vi "TR_DRAW_Trajectory_(offline).vi"(0 "Post-processing parameters":variant, 5 "XY data in":T1=[{"X"=300.0, "Y"=306.0}, {"X"=299.0, "Y"=306.0}, {"X"=295.0, "Y"=297.0}, {"X"=300.0, "Y"=305.0}, {"X"=300.0, "Y"=305.0}, {"X"=299.0, "Y"=306.0}, {"X"=301.0, "Y"=305.0}, {"X"=302.0, "Y"=305.0}, {"X"=299.0, "Y"=306.0}, {"X"=300.0, "Y"=305.0}, {"X"=301.0, "Y"=305.0}, {"X"=300.0, "Y"=305.0}, {"X"=296.0, "Y"=296.0}, {"X"=302.0, "Y"=305.0}, {"X"=300.0, "Y"=305.0}, {"X"=301.0, "Y"=304.0}, {"X"=301.0, "Y"=304.0}, {"X"=301.0, "Y"=304.0}, {"X"=301.0, "Y"=303.0}, {"X"=301.0, "Y"=303.0}, {"X"=301.0, "Y"=303.0}, {"X"=300.0, "Y"=303.0}, {"X"=300.0, "Y"=303.0}, {"X"=301.0, "Y"=303.0}, {"X"=301.0, "Y"=304.0}, {"X"=302.0, "Y"=304.0}, {"X"=303.0, "Y"=304.0}, {"X"=304.0, "Y"=305.0}, {"X"=305.0, "Y"=305.0}, {"X"=306.0, "Y"=305.0}, {"X"=308.0, "Y"=306.0}, {"X"=310.0, "Y"=307.0}, {"X"=311.0, "Y"=309.0}, {"X"=314.0, "Y"=310.0}, {"X"=315.0, "Y"=312.0}, {"X"=318.0, "Y"=315.0}, {"X"=319.0, "Y"=318.0}, {"X"=321.0, "Y"=321.0}, {"X"=323.0, "Y"=324.0}, {"X"=325.0, "Y"=327.0}, {"X"=326.0, "Y"=331.0}, {"X"=327.0, "Y"=335.0}, {"X"=327.0, "Y"=338.0}, {"X"=327.0, "Y"=342.0}, {"X"=326.0, "Y"=347.0}, {"X"=325.0, "Y"=351.0}, {"X"=323.0, "Y"=355.0}, {"X"=321.0, "Y"=360.0}, {"X"=320.0, "Y"=364.0}, {"X"=317.0, "Y"=368.0}, {"X"=315.0, "Y"=372.0}, {"X"=312.0, "Y"=375.0}, {"X"=310.0, "Y"=379.0}, {"X"=308.0, "Y"=382.0}, {"X"=305.0, "Y"=385.0}, {"X"=303.0, "Y"=388.0}, {"X"=299.0, "Y"=391.0}, {"X"=296.0, "Y"=395.0}, {"X"=292.0, "Y"=398.0}, {"X"=287.0, "Y"=401.0}, {"X"=283.0, "Y"=405.0}, {"X"=278.0, "Y"=408.0}, {"X"=273.0, "Y"=411.0}, {"X"=268.0, "Y"=414.0}, {"X"=264.0, "Y"=417.0}, {"X"=259.0, "Y"=419.0}, {"X"=255.0, "Y"=421.0}, {"X"=250.0, "Y"=423.0}, {"X"=246.0, "Y"=424.0}, {"X"=241.0, "Y"=425.0}, {"X"=237.0, "Y"=426.0}, {"X"=232.0, "Y"=426.0}, {"X"=227.0, "Y"=426.0}, {"X"=223.0, "Y"=425.0}, {"X"=219.0, "Y"=425.0}, {"X"=215.0, "Y"=425.0}, {"X"=211.0, "Y"=425.0}, {"X"=209.0, "Y"=425.0}, {"X"=206.0, "Y"=424.0}, {"X"=203.0, "Y"=423.0}, {"X"=200.0, "Y"=421.0}, {"X"=197.0, "Y"=420.0}, {"X"=193.0, "Y"=417.0}, {"X"=189.0, "Y"=414.0}, {"X"=185.0, "Y"=411.0}, {"X"=180.0, "Y"=408.0}, {"X"=175.0, "Y"=406.0}, {"X"=170.0, "Y"=402.0}, {"X"=166.0, "Y"=399.0}, {"X"=161.0, "Y"=395.0}, {"X"=156.0, "Y"=390.0}, {"X"=152.0, "Y"=385.0}, {"X"=148.0, "Y"=379.0}, {"X"=145.0, "Y"=373.0}, {"X"=142.0, "Y"=367.0}, {"X"=140.0, "Y"=359.0}, {"X"=137.0, "Y"=353.0}, {"X"=135.0, "Y"=346.0}, {"X"=134.0, "Y"=339.0}, {"X"=132.0, "Y"=332.0}, {"X"=131.0, "Y"=325.0}, {"X"=131.0, "Y"=318.0}, {"X"=130.0, "Y"=312.0}, {"X"=129.0, "Y"=305.0}, {"X"=128.0, "Y"=299.0}, {"X"=127.0, "Y"=293.0}, {"X"=126.0, "Y"=286.0}, {"X"=125.0, "Y"=279.0}, {"X"=123.0, "Y"=273.0}, {"X"=122.0, "Y"=266.0}, {"X"=120.0, "Y"=259.0}, {"X"=119.0, "Y"=252.0}, {"X"=117.0, "Y"=245.0}, {"X"=116.0, "Y"=239.0}, {"X"=114.0, "Y"=233.0}, {"X"=112.0, "Y"=228.0}, {"X"=111.0, "Y"=223.0}, {"X"=110.0, "Y"=217.0}, {"X"=109.0, "Y"=212.0}, {"X"=108.0, "Y"=206.0}, {"X"=107.0, "Y"=200.0}, {"X"=107.0, "Y"=194.0}, {"X"=107.0, "Y"=187.0}, {"X"=108.0, "Y"=180.0}, {"X"=109.0, "Y"=174.0}, {"X"=110.0, "Y"=167.0}, {"X"=111.0, "Y"=161.0}, {"X"=113.0, "Y"=155.0}, {"X"=115.0, "Y"=149.0}, {"X"=117.0, "Y"=142.0}, {"X"=118.0, "Y"=137.0}, {"X"=120.0, "Y"=131.0}, {"X"=122.0, "Y"=125.0}, {"X"=125.0, "Y"=120.0}, {"X"=127.0, "Y"=114.0}, {"X"=129.0, "Y"=109.0}, {"X"=132.0, "Y"=105.0}, {"X"=135.0, "Y"=100.0}, {"X"=138.0, "Y"=96.0}, {"X"=141.0, "Y"=91.0}, {"X"=145.0, "Y"=87.0}, {"X"=148.0, "Y"=84.0}, {"X"=151.0, "Y"=81.0}, {"X"=154.0, "Y"=78.0}, {"X"=156.0, "Y"=77.0}, {"X"=157.0, "Y"=75.0}, {"X"=160.0, "Y"=73.0}, {"X"=163.0, "Y"=72.0}, {"X"=165.0, "Y"=71.0}, {"X"=167.0, "Y"=70.0}, {"X"=171.0, "Y"=68.0}, {"X"=173.0, "Y"=67.0}, {"X"=176.0, "Y"=66.0}, {"X"=179.0, "Y"=65.0}, {"X"=183.0, "Y"=65.0}, {"X"=187.0, "Y"=64.0}, {"X"=191.0, "Y"=64.0}, {"X"=195.0, "Y"=64.0}, {"X"=198.0, "Y"=64.0}, {"X"=202.0, "Y"=65.0}, {"X"=205.0, "Y"=66.0}, {"X"=209.0, "Y"=67.0}, {"X"=213.0, "Y"=67.0}, {"X"=217.0, "Y"=69.0}, {"X"=221.0, "Y"=70.0}, {"X"=226.0, "Y"=72.0}, {"X"=230.0, "Y"=73.0}, {"X"=236.0, "Y"=75.0}, {"X"=240.0, "Y"=77.0}, {"X"=245.0, "Y"=79.0}, {"X"=249.0, "Y"=82.0}, {"X"=253.0, "Y"=84.0}, {"X"=258.0, "Y"=87.0}, {"X"=262.0, "Y"=89.0}, {"X"=266.0, "Y"=92.0}, {"X"=269.0, "Y"=95.0}, {"X"=274.0, "Y"=98.0}, {"X"=278.0, "Y"=101.0}, {"X"=281.0, "Y"=104.0}, {"X"=285.0, "Y"=107.0}, {"X"=289.0, "Y"=111.0}, {"X"=292.0, "Y"=115.0}, {"X"=296.0, "Y"=118.0}, {"X"=300.0, "Y"=122.0}, {"X"=303.0, "Y"=126.0}, {"X"=307.0, "Y"=130.0}, {"X"=310.0, "Y"=134.0}, {"X"=313.0, "Y"=138.0}, {"X"=316.0, "Y"=142.0}, {"X"=319.0, "Y"=146.0}, {"X"=323.0, "Y"=150.0}, {"X"=326.0, "Y"=155.0}, {"X"=329.0, "Y"=160.0}, {"X"=333.0, "Y"=165.0}, {"X"=336.0, "Y"=170.0}, {"X"=340.0, "Y"=176.0}, {"X"=343.0, "Y"=181.0}, {"X"=346.0, "Y"=186.0}, {"X"=349.0, "Y"=192.0}, {"X"=353.0, "Y"=197.0}, {"X"=356.0, "Y"=202.0}, {"X"=359.0, "Y"=208.0}, {"X"=362.0, "Y"=214.0}, {"X"=364.0, "Y"=220.0}, {"X"=367.0, "Y"=227.0}, {"X"=369.0, "Y"=234.0}, {"X"=372.0, "Y"=242.0}, {"X"=374.0, "Y"=249.0}, {"X"=375.0, "Y"=258.0}, {"X"=377.0, "Y"=266.0}, {"X"=378.0, "Y"=275.0}, {"X"=378.0, "Y"=283.0}, {"X"=379.0, "Y"=291.0}, {"X"=378.0, "Y"=298.0}, {"X"=378.0, "Y"=306.0}, {"X"=377.0, "Y"=314.0}, {"X"=375.0, "Y"=321.0}, {"X"=374.0, "Y"=329.0}, {"X"=372.0, "Y"=337.0}, {"X"=369.0, "Y"=345.0}, {"X"=366.0, "Y"=353.0}, {"X"=363.0, "Y"=361.0}, {"X"=360.0, "Y"=368.0}, {"X"=356.0, "Y"=375.0}, {"X"=353.0, "Y"=382.0}, {"X"=349.0, "Y"=388.0}, {"X"=345.0, "Y"=394.0}, {"X"=341.0, "Y"=400.0}, {"X"=337.0, "Y"=406.0}, {"X"=333.0, "Y"=411.0}, {"X"=328.0, "Y"=417.0}, {"X"=323.0, "Y"=422.0}, {"X"=318.0, "Y"=428.0}, {"X"=312.0, "Y"=433.0}, {"X"=306.0, "Y"=439.0}, {"X"=300.0, "Y"=444.0}, {"X"=293.0, "Y"=448.0}, {"X"=287.0, "Y"=453.0}, {"X"=280.0, "Y"=457.0}, {"X"=273.0, "Y"=461.0}, {"X"=268.0, "Y"=465.0}, {"X"=262.0, "Y"=468.0}, {"X"=255.0, "Y"=472.0}, {"X"=249.0, "Y"=475.0}, {"X"=242.0, "Y"=479.0}, {"X"=235.0, "Y"=482.0}, {"X"=227.0, "Y"=484.0}, {"X"=219.0, "Y"=486.0}, {"X"=211.0, "Y"=486.0}, {"X"=203.0, "Y"=486.0}, {"X"=196.0, "Y"=486.0}, {"X"=190.0, "Y"=485.0}, {"X"=184.0, "Y"=483.0}, {"X"=179.0, "Y"=481.0}, {"X"=175.0, "Y"=477.0}, {"X"=171.0, "Y"=473.0}, {"X"=167.0, "Y"=468.0}, {"X"=163.0, "Y"=462.0}, {"X"=160.0, "Y"=456.0}, {"X"=158.0, "Y"=449.0}, {"X"=156.0, "Y"=441.0}, {"X"=156.0, "Y"=434.0}, {"X"=155.0, "Y"=425.0}, {"X"=155.0, "Y"=416.0}, {"X"=155.0, "Y"=406.0}, {"X"=155.0, "Y"=396.0}, {"X"=154.0, "Y"=385.0}, {"X"=155.0, "Y"=375.0}, {"X"=155.0, "Y"=364.0}, {"X"=155.0, "Y"=354.0}, {"X"=156.0, "Y"=344.0}, {"X"=156.0, "Y"=334.0}, {"X"=157.0, "Y"=324.0}, {"X"=158.0, "Y"=314.0}, {"X"=159.0, "Y"=304.0}, {"X"=159.0, "Y"=293.0}, {"X"=160.0, "Y"=283.0}, {"X"=160.0, "Y"=273.0}, {"X"=160.0, "Y"=263.0}, {"X"=160.0, "Y"=253.0}, {"X"=161.0, "Y"=243.0}, {"X"=162.0, "Y"=234.0}, {"X"=163.0, "Y"=225.0}, {"X"=164.0, "Y"=216.0}, {"X"=165.0, "Y"=207.0}, {"X"=166.0, "Y"=197.0}, {"X"=168.0, "Y"=188.0}, {"X"=170.0, "Y"=179.0}, {"X"=171.0, "Y"=171.0}, {"X"=173.0, "Y"=162.0}, {"X"=175.0, "Y"=153.0}, {"X"=176.0, "Y"=144.0}, {"X"=178.0, "Y"=135.0}, {"X"=179.0, "Y"=127.0}, {"X"=182.0, "Y"=118.0}, {"X"=183.0, "Y"=111.0}, {"X"=185.0, "Y"=104.0}, {"X"=186.0, "Y"=97.0}, {"X"=187.0, "Y"=90.0}, {"X"=188.0, "Y"=83.0}, {"X"=188.0, "Y"=76.0}, {"X"=188.0, "Y"=69.0}, {"X"=188.0, "Y"=62.0}, {"X"=190.0, "Y"=55.0}, {"X"=191.0, "Y"=47.0}, {"X"=193.0, "Y"=40.0}, {"X"=195.0, "Y"=34.0}, {"X"=197.0, "Y"=28.0}, {"X"=199.0, "Y"=22.0}, {"X"=202.0, "Y"=16.0}, {"X"=205.0, "Y"=10.0}, {"X"=207.0, "Y"=5.0}, {"X"=209.0, "Y"=0.0}, {"X"=211.0, "Y"=-5.0}, {"X"=213.0, "Y"=-9.0}, {"X"=217.0, "Y"=-14.0}, {"X"=221.0, "Y"=-18.0}, {"X"=224.0, "Y"=-22.0}, {"X"=226.0, "Y"=-24.0}, {"X"=228.0, "Y"=-26.0}, {"X"=228.0, "Y"=-27.0}, {"X"=228.0, "Y"=-27.0}, {"X"=227.0, "Y"=-27.0}, {"X"=226.0, "Y"=-26.0}, {"X"=227.0, "Y"=-24.0}, {"X"=225.0, "Y"=-22.0}, {"X"=224.0, "Y"=-21.0}, {"X"=225.0, "Y"=-19.0}, {"X"=226.0, "Y"=-16.0}, {"X"=227.0, "Y"=-13.0}, {"X"=229.0, "Y"=-10.0}, {"X"=230.0, "Y"=-5.0}, {"X"=233.0, "Y"=-0.0}, {"X"=238.0, "Y"=4.0}, {"X"=242.0, "Y"=9.0}, {"X"=247.0, "Y"=15.0}, {"X"=252.0, "Y"=21.0}, {"X"=256.0, "Y"=27.0}, {"X"=261.0, "Y"=34.0}, {"X"=266.0, "Y"=41.0}, {"X"=272.0, "Y"=49.0}, {"X"=277.0, "Y"=57.0}, {"X"=282.0, "Y"=65.0}, {"X"=286.0, "Y"=73.0}, {"X"=291.0, "Y"=82.0}, {"X"=296.0, "Y"=90.0}, {"X"=300.0, "Y"=99.0}, {"X"=304.0, "Y"=108.0}, {"X"=307.0, "Y"=118.0}, {"X"=311.0, "Y"=127.0}, {"X"=314.0, "Y"=137.0}, {"X"=318.0, "Y"=147.0}, {"X"=321.0, "Y"=157.0}, {"X"=324.0, "Y"=166.0}, {"X"=326.0, "Y"=175.0}, {"X"=328.0, "Y"=185.0}, {"X"=331.0, "Y"=194.0}, {"X"=333.0, "Y"=204.0}, {"X"=336.0, "Y"=214.0}, {"X"=337.0, "Y"=223.0}, {"X"=339.0, "Y"=233.0}, {"X"=341.0, "Y"=242.0}, {"X"=342.0, "Y"=251.0}, {"X"=343.0, "Y"=260.0}, {"X"=343.0, "Y"=270.0}, {"X"=343.0, "Y"=279.0}, {"X"=343.0, "Y"=287.0}, {"X"=343.0, "Y"=294.0}, {"X"=342.0, "Y"=302.0}, {"X"=341.0, "Y"=310.0}, {"X"=340.0, "Y"=318.0}, {"X"=338.0, "Y"=325.0}, {"X"=335.0, "Y"=332.0}, {"X"=333.0, "Y"=338.0}, {"X"=330.0, "Y"=345.0}, {"X"=328.0, "Y"=351.0}, {"X"=326.0, "Y"=357.0}, {"X"=324.0, "Y"=363.0}, {"X"=322.0, "Y"=369.0}, {"X"=320.0, "Y"=375.0}, {"X"=318.0, "Y"=382.0}, {"X"=315.0, "Y"=388.0}, {"X"=312.0, "Y"=393.0}, {"X"=309.0, "Y"=400.0}, {"X"=306.0, "Y"=406.0}, {"X"=302.0, "Y"=412.0}, {"X"=299.0, "Y"=417.0}, {"X"=295.0, "Y"=423.0}, {"X"=291.0, "Y"=428.0}, {"X"=287.0, "Y"=433.0}, {"X"=283.0, "Y"=438.0}, {"X"=280.0, "Y"=442.0}, {"X"=276.0, "Y"=446.0}, {"X"=272.0, "Y"=450.0}, {"X"=268.0, "Y"=454.0}, {"X"=264.0, "Y"=456.0}, {"X"=260.0, "Y"=458.0}, {"X"=257.0, "Y"=459.0}, {"X"=252.0, "Y"=460.0}, {"X"=248.0, "Y"=460.0}, {"X"=244.0, "Y"=460.0}, {"X"=240.0, "Y"=458.0}, {"X"=235.0, "Y"=456.0}, {"X"=232.0, "Y"=454.0}, {"X"=228.0, "Y"=452.0}, {"X"=225.0, "Y"=449.0}, {"X"=222.0, "Y"=446.0}, {"X"=219.0, "Y"=444.0}, {"X"=216.0, "Y"=442.0}, {"X"=213.0, "Y"=440.0}, {"X"=211.0, "Y"=437.0}, {"X"=209.0, "Y"=434.0}, {"X"=207.0, "Y"=432.0}, {"X"=205.0, "Y"=429.0}, {"X"=203.0, "Y"=425.0}, {"X"=200.0, "Y"=420.0}, {"X"=197.0, "Y"=416.0}, {"X"=194.0, "Y"=411.0}, {"X"=192.0, "Y"=405.0}, {"X"=189.0, "Y"=400.0}, {"X"=187.0, "Y"=394.0}, {"X"=186.0, "Y"=388.0}, {"X"=185.0, "Y"=382.0}, {"X"=185.0, "Y"=376.0}, {"X"=186.0, "Y"=370.0}, {"X"=187.0, "Y"=362.0}, {"X"=189.0, "Y"=354.0}, {"X"=191.0, "Y"=346.0}, {"X"=193.0, "Y"=338.0}, {"X"=195.0, "Y"=329.0}, {"X"=197.0, "Y"=319.0}, {"X"=199.0, "Y"=310.0}, {"X"=202.0, "Y"=300.0}, {"X"=206.0, "Y"=292.0}, {"X"=209.0, "Y"=283.0}, {"X"=213.0, "Y"=275.0}, {"X"=217.0, "Y"=267.0}, {"X"=221.0, "Y"=260.0}, {"X"=225.0, "Y"=252.0}, {"X"=230.0, "Y"=245.0}, {"X"=234.0, "Y"=238.0}, {"X"=239.0, "Y"=232.0}, {"X"=243.0, "Y"=225.0}, {"X"=247.0, "Y"=219.0}, {"X"=252.0, "Y"=213.0}, {"X"=257.0, "Y"=207.0}, {"X"=262.0, "Y"=201.0}, {"X"=267.0, "Y"=196.0}, {"X"=272.0, "Y"=191.0}, {"X"=278.0, "Y"=186.0}, {"X"=283.0, "Y"=182.0}, {"X"=289.0, "Y"=177.0}, {"X"=294.0, "Y"=173.0}, {"X"=299.0, "Y"=169.0}, {"X"=305.0, "Y"=164.0}, {"X"=310.0, "Y"=160.0}, {"X"=315.0, "Y"=155.0}, {"X"=320.0, "Y"=151.0}, {"X"=325.0, "Y"=146.0}, {"X"=329.0, "Y"=142.0}, {"X"=334.0, "Y"=137.0}, {"X"=339.0, "Y"=132.0}, {"X"=344.0, "Y"=129.0}, {"X"=349.0, "Y"=125.0}, {"X"=353.0, "Y"=121.0}, {"X"=358.0, "Y"=117.0}, {"X"=361.0, "Y"=114.0}, {"X"=365.0, "Y"=110.0}, {"X"=369.0, "Y"=106.0}, {"X"=372.0, "Y"=102.0}, {"X"=375.0, "Y"=97.0}, {"X"=378.0, "Y"=92.0}, {"X"=379.0, "Y"=87.0}, {"X"=381.0, "Y"=81.0}, {"X"=383.0, "Y"=76.0}, {"X"=386.0, "Y"=71.0}, {"X"=388.0, "Y"=67.0}, {"X"=390.0, "Y"=63.0}, {"X"=392.0, "Y"=59.0}, {"X"=394.0, "Y"=56.0}, {"X"=395.0, "Y"=53.0}, {"X"=398.0, "Y"=50.0}, {"X"=400.0, "Y"=48.0}, {"X"=402.0, "Y"=46.0}, {"X"=405.0, "Y"=45.0}, {"X"=408.0, "Y"=43.0}, {"X"=410.0, "Y"=43.0}, {"X"=413.0, "Y"=44.0}, {"X"=417.0, "Y"=45.0}, {"X"=421.0, "Y"=49.0}, {"X"=426.0, "Y"=53.0}, {"X"=432.0, "Y"=59.0}, {"X"=436.0, "Y"=66.0}, {"X"=441.0, "Y"=73.0}, {"X"=445.0, "Y"=81.0}, {"X"=448.0, "Y"=89.0}, {"X"=451.0, "Y"=98.0}, {"X"=455.0, "Y"=107.0}, {"X"=457.0, "Y"=116.0}, {"X"=459.0, "Y"=125.0}, {"X"=461.0, "Y"=134.0}, {"X"=462.0, "Y"=143.0}, {"X"=462.0, "Y"=152.0}, {"X"=463.0, "Y"=160.0}, {"X"=463.0, "Y"=170.0}, {"X"=462.0, "Y"=178.0}, {"X"=460.0, "Y"=187.0}, {"X"=459.0, "Y"=196.0}, {"X"=457.0, "Y"=205.0}, {"X"=455.0, "Y"=213.0}, {"X"=453.0, "Y"=221.0}, {"X"=450.0, "Y"=228.0}, {"X"=446.0, "Y"=234.0}, {"X"=443.0, "Y"=239.0}, {"X"=439.0, "Y"=243.0}, {"X"=435.0, "Y"=247.0}, {"X"=432.0, "Y"=250.0}, {"X"=427.0, "Y"=254.0}, {"X"=422.0, "Y"=258.0}, {"X"=417.0, "Y"=262.0}, {"X"=412.0, "Y"=266.0}, {"X"=406.0, "Y"=269.0}, {"X"=400.0, "Y"=272.0}, {"X"=394.0, "Y"=275.0}, {"X"=387.0, "Y"=277.0}, {"X"=381.0, "Y"=279.0}, {"X"=375.0, "Y"=280.0}, {"X"=369.0, "Y"=282.0}, {"X"=363.0, "Y"=282.0}, {"X"=357.0, "Y"=283.0}, {"X"=350.0, "Y"=284.0}, {"X"=344.0, "Y"=284.0}, {"X"=337.0, "Y"=285.0}, {"X"=331.0, "Y"=286.0}, {"X"=324.0, "Y"=288.0}, {"X"=317.0, "Y"=288.0}, {"X"=310.0, "Y"=290.0}, {"X"=304.0, "Y"=291.0}, {"X"=298.0, "Y"=291.0}, {"X"=292.0, "Y"=291.0}, {"X"=286.0, "Y"=291.0}, {"X"=281.0, "Y"=291.0}, {"X"=276.0, "Y"=290.0}, {"X"=271.0, "Y"=289.0}, {"X"=266.0, "Y"=288.0}, {"X"=261.0, "Y"=286.0}, {"X"=257.0, "Y"=284.0}, {"X"=251.0, "Y"=282.0}, {"X"=247.0, "Y"=280.0}, {"X"=243.0, "Y"=278.0}, {"X"=239.0, "Y"=275.0}, {"X"=235.0, "Y"=272.0}, {"X"=232.0, "Y"=269.0}, {"X"=228.0, "Y"=266.0}, {"X"=226.0, "Y"=262.0}, {"X"=223.0, "Y"=259.0}, {"X"=221.0, "Y"=256.0}, {"X"=220.0, "Y"=252.0}, {"X"=218.0, "Y"=249.0}, {"X"=217.0, "Y"=247.0}, {"X"=216.0, "Y"=244.0}, {"X"=215.0, "Y"=242.0}, {"X"=215.0, "Y"=239.0}, {"X"=215.0, "Y"=237.0}, {"X"=216.0, "Y"=234.0}, {"X"=218.0, "Y"=231.0}, {"X"=219.0, "Y"=229.0}, {"X"=221.0, "Y"=227.0}, {"X"=224.0, "Y"=224.0}, {"X"=227.0, "Y"=222.0}, {"X"=230.0, "Y"=221.0}, {"X"=233.0, "Y"=219.0}, {"X"=237.0, "Y"=218.0}, {"X"=241.0, "Y"=216.0}, {"X"=245.0, "Y"=215.0}, {"X"=249.0, "Y"=213.0}, {"X"=253.0, "Y"=212.0}, {"X"=257.0, "Y"=211.0}, {"X"=261.0, "Y"=211.0}, {"X"=265.0, "Y"=210.0}, {"X"=269.0, "Y"=210.0}, {"X"=273.0, "Y"=210.0}, {"X"=276.0, "Y"=210.0}, {"X"=280.0, "Y"=210.0}, {"X"=284.0, "Y"=210.0}, {"X"=287.0, "Y"=211.0}, {"X"=290.0, "Y"=212.0}, {"X"=293.0, "Y"=213.0}, {"X"=296.0, "Y"=215.0}, {"X"=299.0, "Y"=216.0}, {"X"=301.0, "Y"=218.0}, {"X"=303.0, "Y"=220.0}, {"X"=304.0, "Y"=221.0}, {"X"=305.0, "Y"=223.0}, {"X"=306.0, "Y"=225.0}, {"X"=307.0, "Y"=226.0}, {"X"=307.0, "Y"=228.0}, {"X"=307.0, "Y"=229.0}, {"X"=306.0, "Y"=230.0}, {"X"=305.0, "Y"=231.0}, {"X"=304.0, "Y"=232.0}, {"X"=302.0, "Y"=233.0}, {"X"=301.0, "Y"=234.0}, {"X"=299.0, "Y"=234.0}, {"X"=297.0, "Y"=235.0}, {"X"=295.0, "Y"=236.0}, {"X"=293.0, "Y"=237.0}, {"X"=291.0, "Y"=238.0}, {"X"=287.0, "Y"=238.0}, {"X"=284.0, "Y"=238.0}, {"X"=281.0, "Y"=239.0}, {"X"=278.0, "Y"=240.0}, {"X"=274.0, "Y"=241.0}, {"X"=271.0, "Y"=241.0}, {"X"=267.0, "Y"=242.0}, {"X"=264.0, "Y"=243.0}, {"X"=260.0, "Y"=244.0}, {"X"=257.0, "Y"=245.0}, {"X"=254.0, "Y"=246.0}, {"X"=251.0, "Y"=247.0}, {"X"=248.0, "Y"=249.0}, {"X"=245.0, "Y"=251.0}, {"X"=242.0, "Y"=252.0}, {"X"=240.0, "Y"=255.0}, {"X"=237.0, "Y"=258.0}, {"X"=235.0, "Y"=261.0}, {"X"=233.0, "Y"=264.0}, {"X"=231.0, "Y"=268.0}, {"X"=230.0, "Y"=272.0}, {"X"=229.0, "Y"=277.0}, {"X"=228.0, "Y"=281.0}, {"X"=228.0, "Y"=285.0}, {"X"=228.0, "Y"=289.0}, {"X"=228.0, "Y"=293.0}, {"X"=227.0, "Y"=297.0}, {"X"=228.0, "Y"=301.0}, {"X"=228.0, "Y"=304.0}, {"X"=228.0, "Y"=307.0}, {"X"=228.0, "Y"=309.0}, {"X"=228.0, "Y"=311.0}, {"X"=228.0, "Y"=313.0}, {"X"=229.0, "Y"=315.0}, {"X"=229.0, "Y"=316.0}, {"X"=229.0, "Y"=318.0}, {"X"=229.0, "Y"=318.0}, {"X"=230.0, "Y"=319.0}, {"X"=231.0, "Y"=320.0}, {"X"=231.0, "Y"=320.0}, {"X"=232.0, "Y"=320.0}, {"X"=232.0, "Y"=320.0}, {"X"=233.0, "Y"=320.0}, {"X"=233.0, "Y"=320.0}, {"X"=233.0, "Y"=319.0}, {"X"=233.0, "Y"=319.0}, {"X"=233.0, "Y"=319.0}, {"X"=233.0, "Y"=319.0}, {"X"=233.0, "Y"=319.0}, {"X"=233.0, "Y"=319.0}, {"X"=233.0, "Y"=319.0}, {"X"=233.0, "Y"=319.0}, {"X"=233.0, "Y"=319.0}, {"X"=233.0, "Y"=319.0}, {"X"=233.0, "Y"=319.0}, {"X"=233.0, "Y"=319.0}, {"X"=233.0, "Y"=319.0}, {"X"=233.0, "Y"=319.0}, {"X"=233.0, "Y"=319.0}, {"X"=233.0, "Y"=319.0}, {"X"=233.0, "Y"=318.0}, {"X"=233.0, "Y"=317.0}, {"X"=234.0, "Y"=317.0}, {"X"=234.0, "Y"=317.0}, {"X"=235.0, "Y"=317.0}, {"X"=236.0, "Y"=317.0}, {"X"=237.0, "Y"=317.0}, {"X"=238.0, "Y"=316.0}, {"X"=239.0, "Y"=315.0}, {"X"=240.0, "Y"=314.0}, {"X"=241.0, "Y"=312.0}, {"X"=242.0, "Y"=311.0}, {"X"=243.0, "Y"=310.0}, {"X"=244.0, "Y"=309.0}, {"X"=244.0, "Y"=308.0}, {"X"=244.0, "Y"=306.0}, {"X"=244.0, "Y"=305.0}, {"X"=243.0, "Y"=304.0}, {"X"=242.0, "Y"=302.0}, {"X"=240.0, "Y"=301.0}, {"X"=237.0, "Y"=300.0}, {"X"=234.0, "Y"=298.0}, {"X"=231.0, "Y"=297.0}, {"X"=227.0, "Y"=295.0}, {"X"=223.0, "Y"=294.0}, {"X"=219.0, "Y"=292.0}, {"X"=215.0, "Y"=291.0}, {"X"=211.0, "Y"=290.0}, {"X"=206.0, "Y"=289.0}, {"X"=201.0, "Y"=288.0}, {"X"=196.0, "Y"=287.0}, {"X"=191.0, "Y"=286.0}, {"X"=186.0, "Y"=285.0}, {"X"=180.0, "Y"=284.0}, {"X"=175.0, "Y"=283.0}, {"X"=170.0, "Y"=282.0}, {"X"=164.0, "Y"=281.0}, {"X"=159.0, "Y"=280.0}, {"X"=153.0, "Y"=279.0}, {"X"=148.0, "Y"=278.0}, {"X"=143.0, "Y"=278.0}, {"X"=138.0, "Y"=278.0}, {"X"=133.0, "Y"=278.0}, {"X"=129.0, "Y"=278.0}, {"X"=124.0, "Y"=278.0}, {"X"=120.0, "Y"=278.0}, {"X"=115.0, "Y"=278.0}, {"X"=111.0, "Y"=277.0}, {"X"=107.0, "Y"=277.0}, {"X"=103.0, "Y"=276.0}, {"X"=100.0, "Y"=276.0}, {"X"=98.0, "Y"=275.0}, {"X"=96.0, "Y"=275.0}, {"X"=94.0, "Y"=275.0}, {"X"=92.0, "Y"=275.0}, {"X"=91.0, "Y"=275.0}, {"X"=91.0, "Y"=275.0}, {"X"=90.0, "Y"=275.0}, {"X"=90.0, "Y"=275.0}, {"X"=90.0, "Y"=275.0}, {"X"=91.0, "Y"=274.0}, {"X"=91.0, "Y"=274.0}, {"X"=92.0, "Y"=274.0}, {"X"=93.0, "Y"=273.0}, {"X"=94.0, "Y"=273.0}, {"X"=96.0, "Y"=272.0}, {"X"=99.0, "Y"=272.0}, {"X"=102.0, "Y"=272.0}, {"X"=105.0, "Y"=271.0}, {"X"=108.0, "Y"=271.0}, {"X"=112.0, "Y"=270.0}, {"X"=116.0, "Y"=270.0}, {"X"=120.0, "Y"=269.0}, {"X"=125.0, "Y"=268.0}, {"X"=130.0, "Y"=267.0}, {"X"=136.0, "Y"=266.0}, {"X"=142.0, "Y"=265.0}, {"X"=149.0, "Y"=263.0}, {"X"=156.0, "Y"=262.0}, {"X"=163.0, "Y"=261.0}, {"X"=170.0, "Y"=259.0}, {"X"=177.0, "Y"=257.0}, {"X"=184.0, "Y"=255.0}, {"X"=191.0, "Y"=253.0}, {"X"=198.0, "Y"=251.0}, {"X"=204.0, "Y"=249.0}, {"X"=210.0, "Y"=247.0}, {"X"=216.0, "Y"=245.0}, {"X"=221.0, "Y"=243.0}, {"X"=226.0, "Y"=242.0}, {"X"=231.0, "Y"=240.0}, {"X"=235.0, "Y"=239.0}, {"X"=239.0, "Y"=237.0}, {"X"=243.0, "Y"=236.0}, {"X"=245.0, "Y"=235.0}, {"X"=248.0, "Y"=234.0}, {"X"=250.0, "Y"=234.0}, {"X"=252.0, "Y"=233.0}, {"X"=253.0, "Y"=233.0}, {"X"=254.0, "Y"=233.0}, {"X"=255.0, "Y"=233.0}, {"X"=256.0, "Y"=233.0}, {"X"=257.0, "Y"=234.0}, {"X"=257.0, "Y"=234.0}, {"X"=258.0, "Y"=235.0}, {"X"=259.0, "Y"=236.0}, {"X"=259.0, "Y"=236.0}, {"X"=260.0, "Y"=237.0}, {"X"=261.0, "Y"=238.0}, {"X"=261.0, "Y"=239.0}, {"X"=262.0, "Y"=240.0}, {"X"=262.0, "Y"=242.0}, {"X"=262.0, "Y"=243.0}, {"X"=263.0, "Y"=245.0}, {"X"=263.0, "Y"=246.0}, {"X"=263.0, "Y"=246.0}, {"X"=263.0, "Y"=247.0}, {"X"=263.0, "Y"=247.0}, {"X"=264.0, "Y"=247.0}, {"X"=265.0, "Y"=247.0}, {"X"=265.0, "Y"=247.0}, {"X"=267.0, "Y"=247.0}, {"X"=268.0, "Y"=246.0}, {"X"=269.0, "Y"=245.0}, {"X"=271.0, "Y"=244.0}, {"X"=273.0, "Y"=243.0}, {"X"=275.0, "Y"=242.0}, {"X"=277.0, "Y"=241.0}, {"X"=280.0, "Y"=241.0}, {"X"=283.0, "Y"=240.0}, {"X"=285.0, "Y"=240.0}, {"X"=288.0, "Y"=239.0}, {"X"=290.0, "Y"=239.0}, {"X"=292.0, "Y"=239.0}, {"X"=295.0, "Y"=239.0}, {"X"=297.0, "Y"=239.0}, {"X"=299.0, "Y"=239.0}, {"X"=300.0, "Y"=240.0}, {"X"=302.0, "Y"=240.0}, {"X"=303.0, "Y"=240.0}, {"X"=305.0, "Y"=240.0}, {"X"=306.0, "Y"=240.0}, {"X"=306.0, "Y"=240.0}, {"X"=307.0, "Y"=240.0}, {"X"=308.0, "Y"=239.0}, {"X"=309.0, "Y"=238.0}, {"X"=309.0, "Y"=238.0}, {"X"=310.0, "Y"=237.0}, {"X"=310.0, "Y"=237.0}, {"X"=311.0, "Y"=236.0}, {"X"=311.0, "Y"=235.0}, {"X"=311.0, "Y"=234.0}, {"X"=311.0, "Y"=233.0}, {"X"=310.0, "Y"=232.0}, {"X"=309.0, "Y"=231.0}, {"X"=307.0, "Y"=229.0}, {"X"=304.0, "Y"=228.0}, {"X"=302.0, "Y"=226.0}, {"X"=299.0, "Y"=223.0}, {"X"=295.0, "Y"=221.0}, {"X"=292.0, "Y"=219.0}, {"X"=288.0, "Y"=217.0}, {"X"=284.0, "Y"=215.0}, {"X"=280.0, "Y"=213.0}, {"X"=276.0, "Y"=211.0}, {"X"=271.0, "Y"=208.0}, {"X"=267.0, "Y"=206.0}, {"X"=262.0, "Y"=204.0}, {"X"=257.0, "Y"=202.0}, {"X"=251.0, "Y"=200.0}, {"X"=247.0, "Y"=198.0}, {"X"=242.0, "Y"=196.0}, {"X"=237.0, "Y"=194.0}, {"X"=232.0, "Y"=193.0}, {"X"=228.0, "Y"=191.0}, {"X"=224.0, "Y"=188.0}, {"X"=220.0, "Y"=186.0}, {"X"=215.0, "Y"=184.0}, {"X"=211.0, "Y"=181.0}, {"X"=207.0, "Y"=178.0}, {"X"=203.0, "Y"=176.0}, {"X"=198.0, "Y"=173.0}, {"X"=194.0, "Y"=171.0}, {"X"=189.0, "Y"=169.0}, {"X"=185.0, "Y"=168.0}, {"X"=180.0, "Y"=166.0}, {"X"=176.0, "Y"=164.0}, {"X"=171.0, "Y"=162.0}, {"X"=166.0, "Y"=161.0}, {"X"=162.0, "Y"=159.0}, {"X"=159.0, "Y"=158.0}, {"X"=154.0, "Y"=158.0}, {"X"=151.0, "Y"=158.0}, {"X"=147.0, "Y"=158.0}, {"X"=144.0, "Y"=159.0}, {"X"=142.0, "Y"=160.0}, {"X"=140.0, "Y"=161.0}, {"X"=138.0, "Y"=162.0}, {"X"=136.0, "Y"=163.0}, {"X"=135.0, "Y"=164.0}, {"X"=134.0, "Y"=166.0}, {"X"=133.0, "Y"=167.0}, {"X"=131.0, "Y"=169.0}, {"X"=130.0, "Y"=171.0}, {"X"=129.0, "Y"=172.0}, {"X"=127.0, "Y"=174.0}, {"X"=126.0, "Y"=176.0}, {"X"=124.0, "Y"=177.0}, {"X"=123.0, "Y"=178.0}, {"X"=122.0, "Y"=179.0}, {"X"=121.0, "Y"=179.0}, {"X"=120.0, "Y"=179.0}, {"X"=119.0, "Y"=178.0}, {"X"=119.0, "Y"=176.0}, {"X"=118.0, "Y"=174.0}, {"X"=118.0, "Y"=172.0}, {"X"=118.0, "Y"=168.0}, {"X"=119.0, "Y"=165.0}, {"X"=119.0, "Y"=160.0}, {"X"=120.0, "Y"=156.0}, {"X"=121.0, "Y"=151.0}, {"X"=121.0, "Y"=145.0}, {"X"=123.0, "Y"=140.0}, {"X"=124.0, "Y"=134.0}, {"X"=126.0, "Y"=128.0}, {"X"=128.0, "Y"=122.0}, {"X"=131.0, "Y"=117.0}, {"X"=133.0, "Y"=111.0}, {"X"=136.0, "Y"=106.0}, {"X"=139.0, "Y"=100.0}, {"X"=142.0, "Y"=95.0}, {"X"=146.0, "Y"=91.0}, {"X"=149.0, "Y"=87.0}, {"X"=153.0, "Y"=83.0}, {"X"=156.0, "Y"=80.0}, {"X"=159.0, "Y"=79.0}, {"X"=161.0, "Y"=78.0}, {"X"=163.0, "Y"=77.0}, {"X"=165.0, "Y"=77.0}, {"X"=167.0, "Y"=76.0}, {"X"=168.0, "Y"=77.0}, {"X"=169.0, "Y"=77.0}, {"X"=170.0, "Y"=77.0}, {"X"=171.0, "Y"=78.0}, {"X"=172.0, "Y"=79.0}, {"X"=174.0, "Y"=80.0}, {"X"=175.0, "Y"=82.0}, {"X"=177.0, "Y"=84.0}, {"X"=178.0, "Y"=86.0}, {"X"=180.0, "Y"=88.0}, {"X"=182.0, "Y"=92.0}, {"X"=183.0, "Y"=95.0}, {"X"=185.0, "Y"=98.0}, {"X"=188.0, "Y"=102.0}, {"X"=190.0, "Y"=105.0}, {"X"=193.0, "Y"=108.0}, {"X"=196.0, "Y"=111.0}, {"X"=199.0, "Y"=113.0}, {"X"=202.0, "Y"=116.0}, {"X"=205.0, "Y"=118.0}, {"X"=208.0, "Y"=120.0}, {"X"=211.0, "Y"=121.0}, {"X"=214.0, "Y"=123.0}, {"X"=218.0, "Y"=123.0}, {"X"=221.0, "Y"=124.0}, {"X"=224.0, "Y"=124.0}, {"X"=227.0, "Y"=123.0}, {"X"=230.0, "Y"=122.0}, {"X"=233.0, "Y"=120.0}, {"X"=236.0, "Y"=118.0}, {"X"=239.0, "Y"=116.0}, {"X"=241.0, "Y"=114.0}, {"X"=244.0, "Y"=111.0}, {"X"=247.0, "Y"=109.0}, {"X"=250.0, "Y"=107.0}, {"X"=253.0, "Y"=105.0}, {"X"=257.0, "Y"=103.0}, {"X"=259.0, "Y"=100.0}, {"X"=262.0, "Y"=98.0}, {"X"=265.0, "Y"=95.0}, {"X"=268.0, "Y"=93.0}, {"X"=270.0, "Y"=90.0}, {"X"=272.0, "Y"=86.0}, {"X"=274.0, "Y"=83.0}, {"X"=275.0, "Y"=79.0}, {"X"=276.0, "Y"=75.0}, {"X"=277.0, "Y"=71.0}, {"X"=278.0, "Y"=66.0}, {"X"=278.0, "Y"=62.0}, {"X"=278.0, "Y"=58.0}, {"X"=278.0, "Y"=54.0}, {"X"=278.0, "Y"=49.0}, {"X"=278.0, "Y"=45.0}, {"X"=278.0, "Y"=41.0}, {"X"=278.0, "Y"=37.0}, {"X"=277.0, "Y"=33.0}, {"X"=277.0, "Y"=30.0}, {"X"=276.0, "Y"=27.0}, {"X"=276.0, "Y"=24.0}, {"X"=275.0, "Y"=22.0}, {"X"=274.0, "Y"=20.0}, {"X"=273.0, "Y"=18.0}, {"X"=272.0, "Y"=17.0}, {"X"=271.0, "Y"=16.0}, {"X"=270.0, "Y"=15.0}, {"X"=271.0, "Y"=15.0}, {"X"=271.0, "Y"=14.0}, {"X"=271.0, "Y"=14.0}, {"X"=271.0, "Y"=13.0}, {"X"=271.0, "Y"=13.0}, {"X"=271.0, "Y"=12.0}, {"X"=272.0, "Y"=11.0}, {"X"=272.0, "Y"=11.0}, {"X"=272.0, "Y"=10.0}, {"X"=273.0, "Y"=9.0}, {"X"=273.0, "Y"=9.0}, {"X"=273.0, "Y"=8.0}, {"X"=274.0, "Y"=8.0}, {"X"=274.0, "Y"=8.0}, {"X"=275.0, "Y"=7.0}, {"X"=274.0, "Y"=7.0}, {"X"=275.0, "Y"=7.0}, {"X"=275.0, "Y"=7.0}, {"X"=276.0, "Y"=6.0}, {"X"=276.0, "Y"=6.0}, {"X"=276.0, "Y"=6.0}, {"X"=276.0, "Y"=6.0}, {"X"=276.0, "Y"=6.0}, {"X"=276.0, "Y"=5.0}, {"X"=276.0, "Y"=5.0}, {"X"=276.0, "Y"=5.0}, {"X"=276.0, "Y"=5.0}, {"X"=276.0, "Y"=5.0}, {"X"=276.0, "Y"=5.0}, {"X"=276.0, "Y"=5.0}, {"X"=276.0, "Y"=5.0}, {"X"=276.0, "Y"=4.0}, {"X"=277.0, "Y"=4.0}, {"X"=277.0, "Y"=5.0}, {"X"=277.0, "Y"=5.0}, {"X"=277.0, "Y"=5.0}, {"X"=277.0, "Y"=6.0}, {"X"=278.0, "Y"=6.0}, {"X"=277.0, "Y"=6.0}, {"X"=277.0, "Y"=6.0}, {"X"=278.0, "Y"=6.0}, {"X"=277.0, "Y"=7.0}, {"X"=277.0, "Y"=7.0}, {"X"=276.0, "Y"=8.0}, {"X"=274.0, "Y"=9.0}, {"X"=273.0, "Y"=10.0}, {"X"=270.0, "Y"=12.0}, {"X"=268.0, "Y"=14.0}, {"X"=266.0, "Y"=17.0}, {"X"=262.0, "Y"=20.0}, {"X"=259.0, "Y"=24.0}, {"X"=255.0, "Y"=27.0}, {"X"=252.0, "Y"=31.0}, {"X"=249.0, "Y"=35.0}, {"X"=245.0, "Y"=40.0}, {"X"=242.0, "Y"=44.0}, {"X"=239.0, "Y"=49.0}, {"X"=237.0, "Y"=54.0}, {"X"=233.0, "Y"=59.0}, {"X"=230.0, "Y"=65.0}, {"X"=227.0, "Y"=71.0}, {"X"=223.0, "Y"=77.0}, {"X"=220.0, "Y"=83.0}, {"X"=216.0, "Y"=90.0}, {"X"=212.0, "Y"=96.0}, {"X"=208.0, "Y"=102.0}, {"X"=203.0, "Y"=107.0}, {"X"=199.0, "Y"=113.0}, {"X"=194.0, "Y"=118.0}, {"X"=190.0, "Y"=123.0}, {"X"=185.0, "Y"=129.0}, {"X"=180.0, "Y"=134.0}, {"X"=176.0, "Y"=139.0}, {"X"=171.0, "Y"=145.0}, {"X"=167.0, "Y"=151.0}, {"X"=163.0, "Y"=157.0}, {"X"=158.0, "Y"=163.0}, {"X"=154.0, "Y"=168.0}, {"X"=149.0, "Y"=174.0}, {"X"=145.0, "Y"=179.0}, {"X"=142.0, "Y"=183.0}, {"X"=139.0, "Y"=187.0}, {"X"=136.0, "Y"=190.0}, {"X"=133.0, "Y"=193.0}, {"X"=130.0, "Y"=196.0}, {"X"=127.0, "Y"=198.0}, {"X"=124.0, "Y"=200.0}, {"X"=121.0, "Y"=202.0}, {"X"=118.0, "Y"=204.0}, {"X"=114.0, "Y"=205.0}, {"X"=111.0, "Y"=206.0}, {"X"=108.0, "Y"=206.0}, {"X"=104.0, "Y"=206.0}, {"X"=100.0, "Y"=206.0}, {"X"=97.0, "Y"=206.0}, {"X"=94.0, "Y"=206.0}, {"X"=91.0, "Y"=206.0}, {"X"=88.0, "Y"=206.0}, {"X"=85.0, "Y"=207.0}, {"X"=83.0, "Y"=207.0}, {"X"=81.0, "Y"=208.0}, {"X"=79.0, "Y"=209.0}, {"X"=77.0, "Y"=210.0}, {"X"=75.0, "Y"=211.0}, {"X"=74.0, "Y"=212.0}, {"X"=73.0, "Y"=213.0}, {"X"=71.0, "Y"=214.0}, {"X"=71.0, "Y"=215.0}, {"X"=70.0, "Y"=215.0}, {"X"=70.0, "Y"=215.0}, {"X"=70.0, "Y"=216.0}, {"X"=69.0, "Y"=216.0}, {"X"=69.0, "Y"=217.0}, {"X"=69.0, "Y"=217.0}, {"X"=69.0, "Y"=216.0}, {"X"=70.0, "Y"=215.0}, {"X"=70.0, "Y"=214.0}, {"X"=71.0, "Y"=213.0}, {"X"=71.0, "Y"=212.0}, {"X"=72.0, "Y"=210.0}, {"X"=73.0, "Y"=209.0}, {"X"=73.0, "Y"=207.0}, {"X"=74.0, "Y"=205.0}, {"X"=75.0, "Y"=203.0}, {"X"=77.0, "Y"=200.0}, {"X"=79.0, "Y"=197.0}, {"X"=81.0, "Y"=194.0}, {"X"=84.0, "Y"=191.0}, {"X"=86.0, "Y"=188.0}, {"X"=89.0, "Y"=185.0}, {"X"=92.0, "Y"=182.0}, {"X"=95.0, "Y"=179.0}, {"X"=98.0, "Y"=176.0}, {"X"=101.0, "Y"=173.0}, {"X"=104.0, "Y"=170.0}, {"X"=107.0, "Y"=168.0}, {"X"=110.0, "Y"=165.0}, {"X"=113.0, "Y"=163.0}, {"X"=115.0, "Y"=161.0}, {"X"=119.0, "Y"=159.0}, {"X"=121.0, "Y"=157.0}, {"X"=123.0, "Y"=155.0}, {"X"=126.0, "Y"=152.0}, {"X"=129.0, "Y"=150.0}, {"X"=132.0, "Y"=148.0}, {"X"=134.0, "Y"=146.0}, {"X"=137.0, "Y"=144.0}, {"X"=139.0, "Y"=143.0}, {"X"=140.0, "Y"=141.0}, {"X"=142.0, "Y"=140.0}, {"X"=144.0, "Y"=139.0}, {"X"=146.0, "Y"=137.0}, {"X"=148.0, "Y"=134.0}, {"X"=151.0, "Y"=132.0}, {"X"=154.0, "Y"=130.0}, {"X"=157.0, "Y"=127.0}, {"X"=161.0, "Y"=124.0}, {"X"=164.0, "Y"=121.0}, {"X"=168.0, "Y"=117.0}, {"X"=172.0, "Y"=113.0}, {"X"=176.0, "Y"=110.0}, {"X"=179.0, "Y"=106.0}, {"X"=183.0, "Y"=102.0}, {"X"=187.0, "Y"=98.0}, {"X"=191.0, "Y"=95.0}, {"X"=194.0, "Y"=92.0}, {"X"=198.0, "Y"=89.0}, {"X"=201.0, "Y"=86.0}, {"X"=205.0, "Y"=83.0}, {"X"=209.0, "Y"=81.0}, {"X"=213.0, "Y"=79.0}, {"X"=217.0, "Y"=76.0}, {"X"=221.0, "Y"=75.0}, {"X"=225.0, "Y"=73.0}, {"X"=229.0, "Y"=71.0}, {"X"=232.0, "Y"=70.0}, {"X"=236.0, "Y"=69.0}, {"X"=238.0, "Y"=68.0}, {"X"=241.0, "Y"=67.0}, {"X"=243.0, "Y"=66.0}, {"X"=246.0, "Y"=65.0}, {"X"=248.0, "Y"=64.0}, {"X"=251.0, "Y"=63.0}, {"X"=253.0, "Y"=61.0}, {"X"=257.0, "Y"=60.0}, {"X"=260.0, "Y"=58.0}, {"X"=263.0, "Y"=56.0}, {"X"=267.0, "Y"=55.0}, {"X"=269.0, "Y"=53.0}, {"X"=272.0, "Y"=51.0}, {"X"=274.0, "Y"=50.0}, {"X"=276.0, "Y"=47.0}, {"X"=279.0, "Y"=45.0}, {"X"=281.0, "Y"=44.0}, {"X"=282.0, "Y"=42.0}, {"X"=284.0, "Y"=41.0}, {"X"=285.0, "Y"=39.0}, {"X"=287.0, "Y"=38.0}, {"X"=288.0, "Y"=37.0}, {"X"=289.0, "Y"=36.0}, {"X"=290.0, "Y"=35.0}, {"X"=292.0, "Y"=35.0}, {"X"=293.0, "Y"=35.0}, {"X"=294.0, "Y"=35.0}, {"X"=294.0, "Y"=35.0}, {"X"=294.0, "Y"=36.0}, {"X"=293.0, "Y"=37.0}, {"X"=292.0, "Y"=38.0}, {"X"=291.0, "Y"=39.0}, {"X"=290.0, "Y"=41.0}, {"X"=290.0, "Y"=43.0}, {"X"=289.0, "Y"=44.0}, {"X"=288.0, "Y"=46.0}, {"X"=286.0, "Y"=48.0}, {"X"=285.0, "Y"=50.0}, {"X"=284.0, "Y"=52.0}, {"X"=282.0, "Y"=54.0}, {"X"=280.0, "Y"=56.0}, {"X"=278.0, "Y"=58.0}, {"X"=276.0, "Y"=60.0}, {"X"=274.0, "Y"=62.0}, {"X"=272.0, "Y"=64.0}, {"X"=269.0, "Y"=66.0}, {"X"=266.0, "Y"=68.0}, {"X"=264.0, "Y"=69.0}, {"X"=261.0, "Y"=71.0}, {"X"=258.0, "Y"=73.0}, {"X"=254.0, "Y"=75.0}, {"X"=251.0, "Y"=78.0}, {"X"=248.0, "Y"=80.0}, {"X"=245.0, "Y"=83.0}, {"X"=241.0, "Y"=86.0}, {"X"=238.0, "Y"=89.0}, {"X"=234.0, "Y"=92.0}, {"X"=230.0, "Y"=96.0}, {"X"=226.0, "Y"=100.0}, {"X"=222.0, "Y"=103.0}, {"X"=218.0, "Y"=107.0}, {"X"=214.0, "Y"=110.0}, {"X"=211.0, "Y"=113.0}, {"X"=207.0, "Y"=115.0}, {"X"=202.0, "Y"=118.0}, {"X"=198.0, "Y"=121.0}, {"X"=194.0, "Y"=122.0}, {"X"=191.0, "Y"=124.0}, {"X"=187.0, "Y"=126.0}, {"X"=183.0, "Y"=128.0}, {"X"=179.0, "Y"=129.0}, {"X"=176.0, "Y"=130.0}, {"X"=173.0, "Y"=130.0}, {"X"=169.0, "Y"=130.0}, {"X"=166.0, "Y"=131.0}, {"X"=163.0, "Y"=131.0}, {"X"=160.0, "Y"=131.0}, {"X"=157.0, "Y"=131.0}, {"X"=154.0, "Y"=131.0}, {"X"=153.0, "Y"=132.0}, {"X"=150.0, "Y"=133.0}, {"X"=148.0, "Y"=133.0}, {"X"=145.0, "Y"=135.0}, {"X"=143.0, "Y"=136.0}, {"X"=140.0, "Y"=137.0}, {"X"=138.0, "Y"=139.0}, {"X"=135.0, "Y"=141.0}, {"X"=132.0, "Y"=143.0}, {"X"=129.0, "Y"=145.0}, {"X"=126.0, "Y"=147.0}, {"X"=123.0, "Y"=150.0}, {"X"=120.0, "Y"=152.0}, {"X"=117.0, "Y"=155.0}, {"X"=114.0, "Y"=158.0}, {"X"=112.0, "Y"=161.0}, {"X"=109.0, "Y"=164.0}, {"X"=106.0, "Y"=167.0}, {"X"=103.0, "Y"=170.0}, {"X"=101.0, "Y"=173.0}, {"X"=99.0, "Y"=176.0}, {"X"=97.0, "Y"=178.0}, {"X"=95.0, "Y"=180.0}, {"X"=93.0, "Y"=183.0}, {"X"=91.0, "Y"=185.0}, {"X"=89.0, "Y"=187.0}, {"X"=88.0, "Y"=190.0}, {"X"=87.0, "Y"=192.0}, {"X"=85.0, "Y"=193.0}, {"X"=84.0, "Y"=196.0}, {"X"=83.0, "Y"=198.0}, {"X"=82.0, "Y"=200.0}, {"X"=81.0, "Y"=201.0}, {"X"=79.0, "Y"=204.0}, {"X"=78.0, "Y"=205.0}, {"X"=77.0, "Y"=206.0}, {"X"=77.0, "Y"=207.0}, {"X"=76.0, "Y"=208.0}, {"X"=76.0, "Y"=208.0}, {"X"=75.0, "Y"=208.0}, {"X"=74.0, "Y"=209.0}, {"X"=74.0, "Y"=208.0}, {"X"=74.0, "Y"=207.0}, {"X"=73.0, "Y"=208.0}, {"X"=73.0, "Y"=207.0}, {"X"=73.0, "Y"=206.0}, {"X"=72.0, "Y"=206.0}, {"X"=73.0, "Y"=206.0}, {"X"=73.0, "Y"=205.0}, {"X"=74.0, "Y"=204.0}, {"X"=74.0, "Y"=203.0}, {"X"=74.0, "Y"=203.0}, {"X"=75.0, "Y"=202.0}, {"X"=75.0, "Y"=202.0}, {"X"=76.0, "Y"=201.0}, {"X"=76.0, "Y"=200.0}, {"X"=76.0, "Y"=200.0}, {"X"=77.0, "Y"=199.0}, {"X"=77.0, "Y"=199.0}, {"X"=77.0, "Y"=199.0}, {"X"=78.0, "Y"=199.0}, {"X"=78.0, "Y"=199.0}, {"X"=78.0, "Y"=199.0}, {"X"=78.0, "Y"=199.0}, {"X"=79.0, "Y"=199.0}, {"X"=80.0, "Y"=198.0}, {"X"=80.0, "Y"=198.0}, {"X"=80.0, "Y"=198.0}, {"X"=81.0, "Y"=198.0}, {"X"=81.0, "Y"=198.0}, {"X"=81.0, "Y"=198.0}, {"X"=82.0, "Y"=197.0}, {"X"=83.0, "Y"=198.0}, {"X"=83.0, "Y"=198.0}, {"X"=84.0, "Y"=198.0}, {"X"=85.0, "Y"=198.0}, {"X"=86.0, "Y"=198.0}, {"X"=86.0, "Y"=198.0}, {"X"=87.0, "Y"=198.0}, {"X"=88.0, "Y"=198.0}, {"X"=88.0, "Y"=198.0}, {"X"=89.0, "Y"=197.0}, {"X"=90.0, "Y"=197.0}, {"X"=92.0, "Y"=196.0}, {"X"=93.0, "Y"=194.0}, {"X"=93.0, "Y"=194.0}, {"X"=94.0, "Y"=193.0}, {"X"=96.0, "Y"=191.0}, {"X"=97.0, "Y"=190.0}, {"X"=98.0, "Y"=188.0}, {"X"=99.0, "Y"=188.0}, {"X"=100.0, "Y"=187.0}, {"X"=101.0, "Y"=185.0}, {"X"=102.0, "Y"=184.0}, {"X"=103.0, "Y"=183.0}, {"X"=104.0, "Y"=181.0}, {"X"=104.0, "Y"=180.0}, {"X"=105.0, "Y"=179.0}, {"X"=106.0, "Y"=178.0}, {"X"=107.0, "Y"=177.0}, {"X"=108.0, "Y"=176.0}, {"X"=108.0, "Y"=175.0}, {"X"=109.0, "Y"=175.0}, {"X"=110.0, "Y"=174.0}, {"X"=110.0, "Y"=173.0}, {"X"=110.0, "Y"=173.0}, {"X"=110.0, "Y"=172.0}, {"X"=110.0, "Y"=172.0}, {"X"=110.0, "Y"=172.0}, {"X"=111.0, "Y"=171.0}, {"X"=111.0, "Y"=170.0}, {"X"=111.0, "Y"=170.0}, {"X"=112.0, "Y"=169.0}, {"X"=112.0, "Y"=168.0}, {"X"=113.0, "Y"=168.0}, {"X"=112.0, "Y"=167.0}, {"X"=113.0, "Y"=166.0}, {"X"=113.0, "Y"=166.0}, {"X"=113.0, "Y"=166.0}, {"X"=113.0, "Y"=166.0}, {"X"=112.0, "Y"=166.0}, {"X"=112.0, "Y"=165.0}, {"X"=112.0, "Y"=165.0}, {"X"=111.0, "Y"=165.0}, {"X"=111.0, "Y"=164.0}, {"X"=111.0, "Y"=164.0}, {"X"=111.0, "Y"=164.0}, {"X"=111.0, "Y"=164.0}, {"X"=111.0, "Y"=165.0}, {"X"=111.0, "Y"=165.0}, {"X"=110.0, "Y"=165.0}, {"X"=110.0, "Y"=165.0}, {"X"=110.0, "Y"=166.0}, {"X"=110.0, "Y"=166.0}, {"X"=110.0, "Y"=166.0}, {"X"=110.0, "Y"=166.0}, {"X"=110.0, "Y"=166.0}, {"X"=110.0, "Y"=166.0}, {"X"=110.0, "Y"=166.0}, {"X"=110.0, "Y"=166.0}, {"X"=109.0, "Y"=167.0}, {"X"=109.0, "Y"=167.0}, {"X"=109.0, "Y"=168.0}, {"X"=109.0, "Y"=168.0}, {"X"=109.0, "Y"=169.0}, {"X"=108.0, "Y"=169.0}, {"X"=108.0, "Y"=170.0}, {"X"=108.0, "Y"=170.0}, {"X"=108.0, "Y"=170.0}, {"X"=108.0, "Y"=170.0}, {"X"=108.0, "Y"=170.0}, {"X"=109.0, "Y"=170.0}, {"X"=109.0, "Y"=170.0}, {"X"=109.0, "Y"=170.0}, {"X"=110.0, "Y"=169.0}, {"X"=111.0, "Y"=169.0}, {"X"=112.0, "Y"=168.0}], 7 "Track start, s":dbl=-1.0 format="%#_13g", 9 "Track finish, s":dbl=-1.0 format="%#_13g", 11 "Error In":errorcluster) -> (4 "Overlays cluster out":T2, 6 "XY data out":T1, 15 "Error Out":errorcluster)   [LabVIEW 2018, in "Tracks Repair.lvlib"]
uses:
  Tracks Repair.lvlib
  SubVi's/Controls/CTL_Overlays_cluster.ctl
  SubVi's/Controls/CTL_Full_Track_Array.ctl
  SubVi's/Controls/CTL_Post-processing_params.ctl
  SubVi's/Controls/CTL_Filter_selector.ctl
  SubVi's/Controls/CTL_Mouse_Draw_Params.ctl
  <vilib>/vision/Image Controls.llb/IMAQ Image.ctl
  SubVi's/Controls/CTL_Calibration_parameters.ctl
  SubVi's/Controls/CTL_Dispenser_calibration_info.ctl
  SubVi's/Controls/CTL_Pixel_to_Zone_array.ctl
  Tracker.lvlib
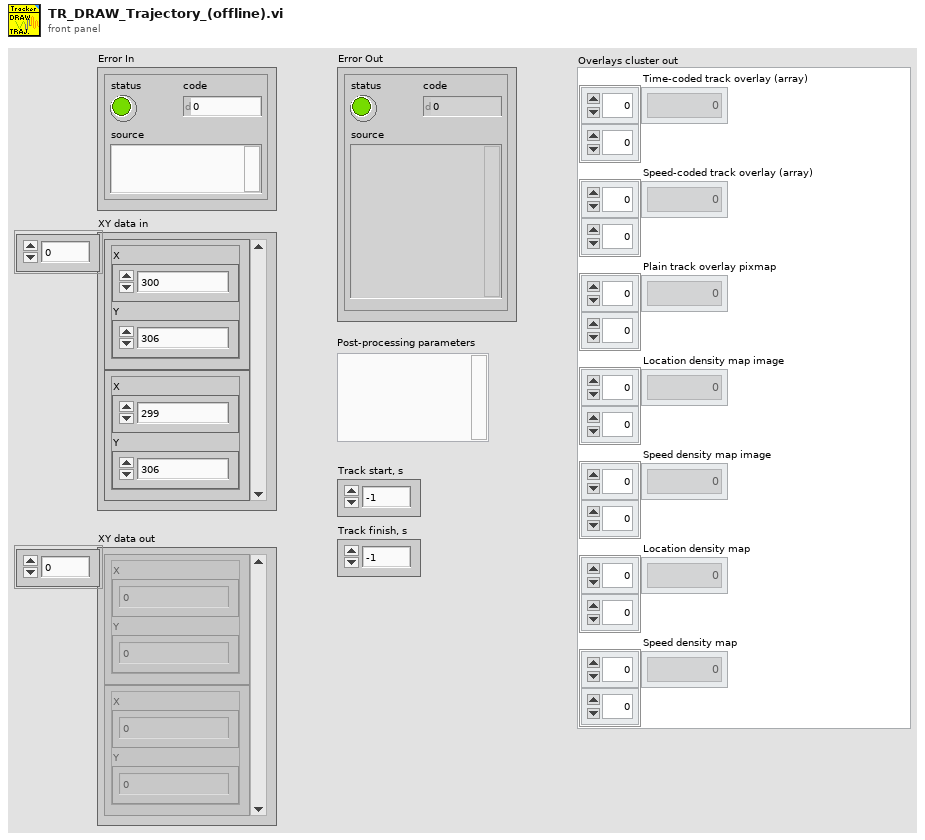
[diagram p1: front panel]
types:
  T1 = typedef "Tracker.lvlib/CTL_Full_Track_Array.ctl" = cluster{"X":dbl, "Y":dbl}[]
  T2 = typedef "Tracker.lvlib/CTL_Overlays_cluster.ctl" = cluster{"Time-coded track overlay (array)":u32[][], "Speed-coded track overlay (array)":u32[][], "Plain track overlay pixmap":u32[][], "Location density map image":u32[][], "Speed density map image":u32[][], "Location density map":dbl[][], "Speed density map":dbl[][]}
  T3 = typedef "Tracker.lvlib/CTL_Post-processing_params.ctl" = cluster{"Defragment TDMS? (F)":bool, "Start time (SW)":timestamp, "Start time (HW)":u32, "Data filtering":T4, "Mouse drawing parameters":T5, "Size of the image (480x480)":cluster{"X size":dbl, "Y size":dbl}, "Image ref. in":T6, "Calibration parameters":T7, "Pixel to zone":T9}
  T4 = typedef "Tracker.lvlib/CTL_Filter_selector.ctl" = cluster{"Filter type":enum16{"None", "Savitzky-Golay"}, "Length":i32, "Order":i32}
  T5 = typedef "Tracker.lvlib/CTL_Mouse_Draw_Params.ctl" = cluster{"Trace length, samples":u16, "Rainbow track":bool, "Rainbow track is speed":bool, "Bright mouse lineout":bool, "Colors array":u32[], "Pixels per mm":dbl}
  T6 = typedef "IMAQ Image.ctl" = refnum<image>
  T7 = typedef "Tracker.lvlib/CTL_Calibration_parameters.ctl" = cluster{"Timing calibration sw/hw":dbl, "True FPS":dbl, "True frame time, s":dbl, "Disp. calibration info":T8}
  T8 = typedef "Tracker.lvlib/CTL_Dispenser_calibration_info.ctl" = cluster{"Channel":u8, "Speed, µl per ms":dbl}[]
  T9 = typedef "Tracker.lvlib/CTL_Pixel_to_Zone_array.ctl" = i8[][]
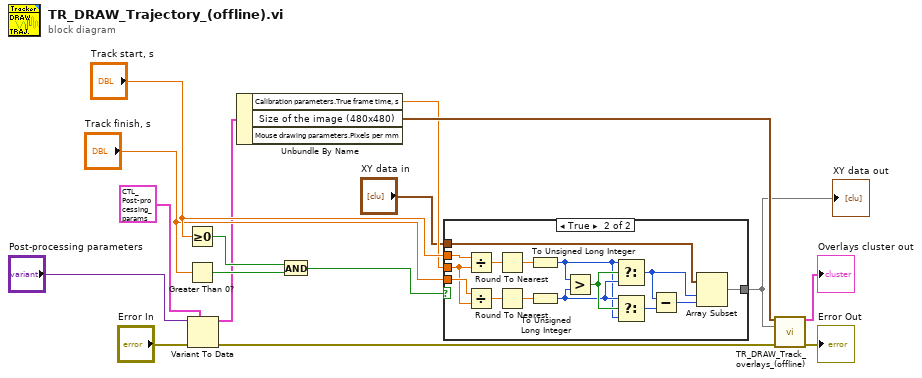
[diagram p0: block diagram]
diagram:
  n1 = Greater Or Equal To 0?(x="Track start, s") -> (x >= 0?=w11:bool)
  n2 = Greater Than 0?(x="Track finish, s") -> (x > 0?=w12:bool)
  n3 = Variant To Data(error in="Error In", type=T3 {"Defragment TDMS? (F)"=FALSE, "Start time (SW)"=timestamp(0 s since 1904-01-01), "Start time (HW)"=0, "Data filtering"={"Filter type"=enum."Savitzky-Golay", "Length"=41, "Order"=3}, "Mouse drawing parameters"={"Trace length, samples"=0, "Rainbow track"=FALSE, "Rainbow track is speed"=FALSE, "Bright mouse lineout"=FALSE, "Colors array"=[], "Pixels per mm"=0.0}, "Size of the image (480x480)"={"X size"=480.0, "Y size"=480.0}, "Image ref. in"=refnum, "Calibration parameters"={"Timing calibration sw/hw"=1.0, "True FPS"=80.0, "True frame time, s"=0.0125, "Disp. calibration info"=[]}, "Pixel to zone"=[]} ("Processing parameters"), Variant="Post-processing parameters") -> (data=w4:T3, error out=w2:errorcluster)
  n4 = Unbundle By Name(w4) -> ("Calibration parameters.True frame time, s"=w7:dbl, "Size of the image (480x480)"=w16:cluster{"X size":dbl, "Y size":dbl})  [unwired: 1 out]
  n5 = And(x=w11, y=w12) -> (x .and. y?=w10:bool)
  n6 = case shown="True" w10 {
    tunnel: "Track start, s" -> [_ w32]
    tunnel: "Track finish, s" -> [_ w31]
    tunnel: w7 -> [_ w30]
    tunnel: "XY data in" -> [w17 w25]
    tunnel: [w17 w24] -> w14
    frame False {
    }
    frame True {
      n7 = Divide(x=w32, y=w30) -> (x/y=w29:dbl)
      n8 = Divide(x=w31, y=w30) -> (x/y=w28:dbl)
      n9 = Round To Nearest(number=w29) -> (nearest integer value=w27:dbl)
      n10 = Round To Nearest(number=w28) -> (nearest integer value=w26:dbl)
      n11 = To Unsigned Long Integer(number=w27) -> (unsigned 32bit integer=w18:u32)
      n12 = To Unsigned Long Integer(number=w26) -> (unsigned 32bit integer=w19:u32)
      n13 = Greater?(x=w18, y=w19) -> (0:w22:bool)
      n14 = Select(t=w18, s=w22, f=w19) -> (s? t:f=w21:u32)
      n15 = Select(t=w19, s=w22, f=w18) -> (s? t:f=w20:u32)
      n16 = Subtract(x=w21, y=w20) -> (x-y=w23:u32)
      n17 = Array Subset(array=w25, index=w21, length=w23) -> (w24:T1)
    }
  }
  "XY data out" <- w14
  n18 = call "TR_DRAW_Track_overlays_(offline).vi"("Image size"=w16, "Full track array"=w14, "Error In"=w2) -> ("Overlays cluster out"=→"Overlays cluster out":T2, "Error Out"=→"Error Out":errorcluster)  [unwired: 11 in]
